vi "Accelration Control (by Throttle).vi"(2 "acc":dbl, 3 "Yinput":dbl, 4 "Xinput":dbl) -> (0 "Youtput":dbl format="%.2f", 1 "Xoutput":dbl format="%.2f")   [LabVIEW 2012]
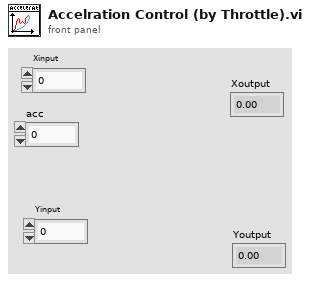
[diagram p1: front panel]
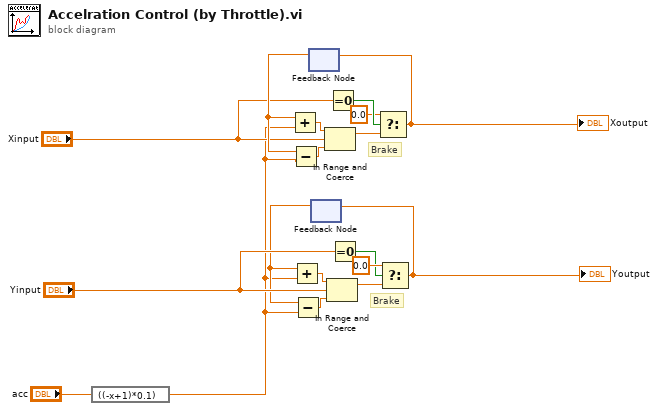
[diagram p0: block diagram]
diagram:
  # "Brake"
  # "Brake"
  n1 = expression code="((-x+1)*0.1)"("acc") -> (w1:dbl)
  n2 = feedback #1() -> (w16:dbl)  [unwired: 1 in]
  n3 = Add(x=w16, y=w1) -> (x+y=w17:dbl)
  n4 = Subtract(x=w16, y=w1) -> (x-y=w18:dbl)
  n5 = feedback #2() -> (w4:dbl)  [unwired: 1 in]
  n6 = Add(x=w4, y=w1) -> (x+y=w3:dbl)
  n7 = Subtract(x=w4, y=w1) -> (x-y=w2:dbl)
  n8 = In Range and Coerce(upper limit=w17, x="Xinput", lower limit=w18) -> (coerced(x)=w12:dbl)  [unwired: 1 out]
  n9 = In Range and Coerce(upper limit=w3, x="Yinput", lower limit=w2) -> (coerced(x)=w7:dbl)  [unwired: 1 out]
  n10 = Equal To 0?(x="Xinput") -> (x = 0?=w13:bool)
  n11 = Equal To 0?(x="Yinput") -> (x = 0?=w6:bool)
  n12 = Select(t=0.0, s=w13, f=w12) -> (s? t:f=w10:dbl)
  "Xoutput" <- w10
  n13 = feedback-in #1(w10) -> ()
  n14 = Select(t=0.0, s=w6, f=w7) -> (s? t:f=w9:dbl)
  "Youtput" <- w9
  n15 = feedback-in #2(w9) -> ()
